vi "改变数字字符串精度.vi"(0 "字符串":string, 1 "精度位数":u32) -> (2 "是否未数字":bool, 3 "输出字符串":string)   [LabVIEW 2014]
doc: "该模板用于创建子VI。"
panel:
  out "error out":errorcluster caption="错误输出"
  in  "error in (no error)":errorcluster caption="错误输入（无错误）"
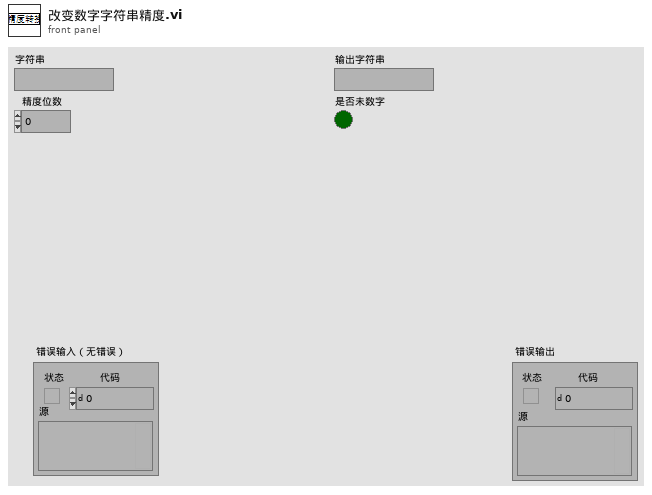
[diagram p1: front panel]
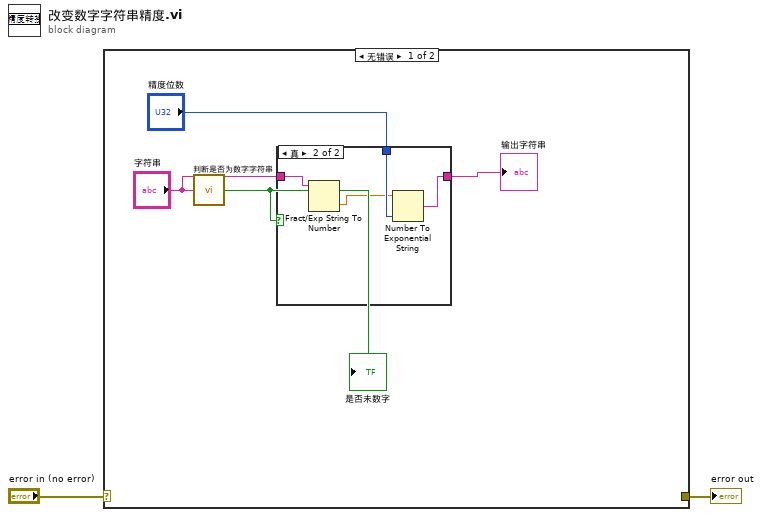
[diagram p0: block diagram]
diagram:
  n1 = case shown="无错误" "error in (no error)" {
    selector: "error in (no error)" -> [_ w12]
    tunnel: [_ w12] -> w1
    frame No Error {
      n2 = call "判断是否为数字字符串.vi"("字符串"="字符串") -> ("是否为数字"=w6:bool)
      "是否未数字" <- w6
      n3 = case shown="真" w6 {
        tunnel: "字符串" -> [w7 w11]
        tunnel: [w7 w9] -> w4
        tunnel: "精度位数" -> [_ w10]
        frame False {
        }
        frame True {
          n4 = Fract/Exp String To Number(string=w11) -> (number=w8:dbl)  [unwired: 3 in, 1 out]
          n5 = Number To Exponential String(number=w8, precision (6)=w10) -> (E-format string=w9:string)  [unwired: 2 in]
        }
      }
      "输出字符串" <- w4
    }
    frame Error {
    }
  }
  "error out" <- w1
